vi "Open IPF.vi"(3 "Error In":errorcluster, 4 "?":T2) -> (0 "Error Out":errorcluster, 1 "IPF refnum":T1, 2 "IPF Path":path)   [LabVIEW 2018]
uses:
  Type Defs/Open IPF.ctl
  <vilib>/Utility/config.llb/Config Data RefNum.ctl
  <vilib>/Utility/config.llb/NI_LVConfig.lvlib
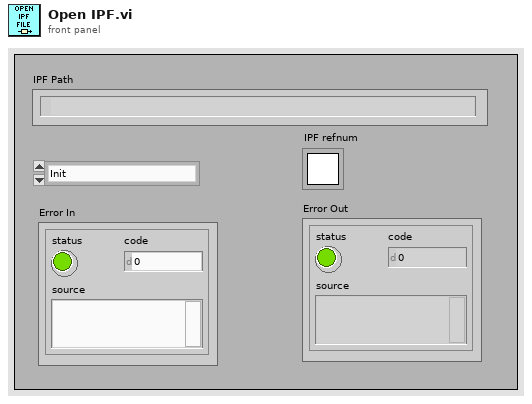
[diagram p1: front panel]
types:
  T1 = typedef "NI_LVConfig.lvlib/Config Data RefNum.ctl" = refnum<k1>
  T2 = typedef "Open IPF.ctl" = enum16{"Init", "Create IPF"}
  T3 = enum32{"existing file", "new file", "new or existing file", "existing dir", "new dir", "new or existing dir", "existing file (use LLBs)", "new file (use LLBs)", "new or existing file (use LLBs)", "new or existing file or directory (use LLBs)"}
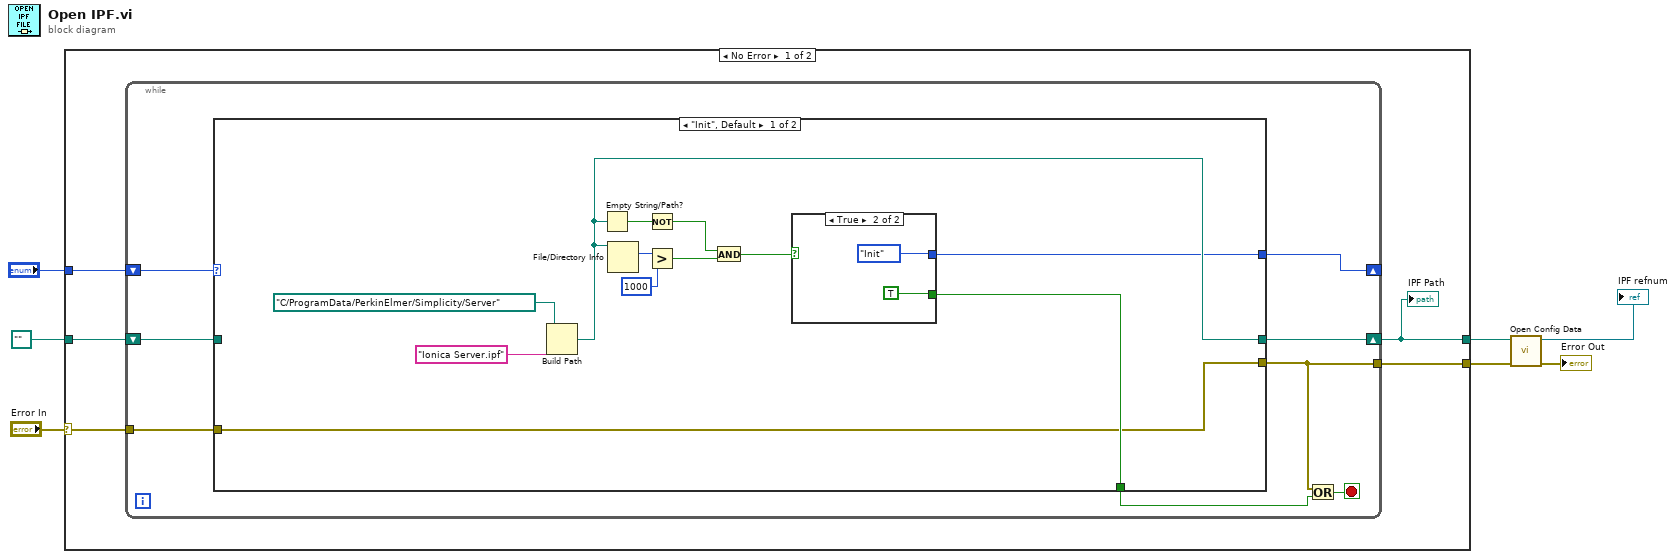
[diagram p0: block diagram]
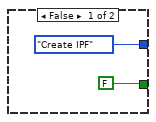
[diagram p2: hidden frame]
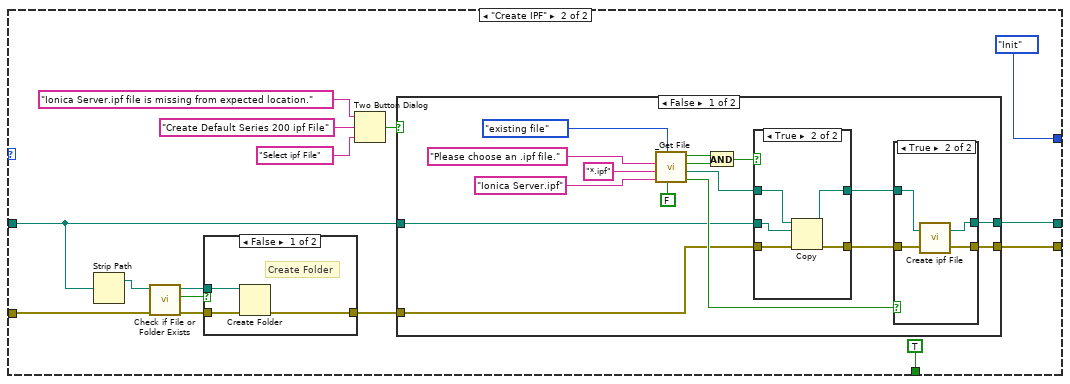
[diagram p3: hidden frame]
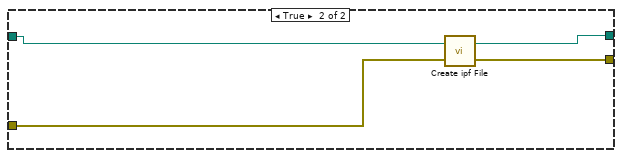
[diagram p6: hidden frame]
diagram:
  n1 = case shown="No Error" "Error In" {
    selector: "Error In" -> [w11 w90]
    tunnel: [w10 w90] -> w5
    tunnel: "?" -> [w12 _]
    tunnel: [w8 w89] -> w4
    tunnel: path "" ("ipf file path") -> [w9 w89]
    frame No Error {
      n2 = while {
        tunnel: w11 -> [w19]
        tunnel: [w15] -> w10
        shift-right: [w17] -> w8
        shift-left: w9 -> [w18]
        shift-right: [w13] -> _
        shift-left: w12 -> [w20]
        stop <- w16 stop-if-true
        n3 = case shown="\"Init\", Default" w20 {
          tunnel: w19 -> [w21 w44]
          tunnel: [w21 w39] -> w15
          tunnel: w18 -> [_ w42]
          tunnel: [w25 w40] -> w17
          tunnel: [w23 TRUE] -> w14
          tunnel: [w22 Open_IPF."Init"] -> w13
          frame "Init", Default {
            n4 = Build Path(base path=path "C:/ProgramData/PerkinElmer/Simplicity/Server" ("appended path"), name or relative path="Ionica Server.ipf") -> (appended path=w25:path)
            n5 = Empty String/Path?(string/path=w25) -> (empty?=w28:bool)
            n6 = File/Directory Info(path=w25) -> (size=w29:i64)  [unwired: 1 in, 6 out]
            n7 = Not(x=w28) -> (.not. x?=w26:bool)
            n8 = Greater?(x=w29, y=i64 1000) -> (0:w27:bool)
            n9 = And(x=w26, y=w27) -> (x .and. y?=w24:bool)
            n10 = case shown="True" w24 {
              tunnel: [FALSE TRUE] -> w23
              tunnel: [Open_IPF."Create IPF" Open_IPF."Init"] -> w22
              frame False {
              }
              frame True {
              }
            }
          }
          frame "Create IPF" {
            n11 = Strip Path(path=w42) -> (stripped path=w48:path)  [unwired: 1 out]
            n12 = call <vilib>:"Check if File or Folder Exists.vi"("error in (no error)"=w44, "path"=w48) -> ("error out"=w51:errorcluster, "file or folder exists?"=w49:bool, "dup path"=w50:path)  [unwired: 7 in]
            n13 = case shown="False" w49 {
              tunnel: w51 -> [w87 w88]
              tunnel: [w86 w88] -> w43
              tunnel: w50 -> [w85 _]
              frame False {
                # "Create Folder"
                n14 = Create Folder(path (use dialog)=w85, error in=w87) -> (error out=w86:errorcluster)  [unwired: 1 in, 2 out]
              }
              frame True {
              }
            }
            n15 = Two Button Dialog(message="Ionica Server.ipf file is missing from expected location.", 1:"Select ipf File" ("T button name (\"OK\")"), 2:"Create Default Series 200 ipf File" ("T button name (\"OK\")")) -> (T button?=w41:bool)
            n16 = case shown="False" w41 {
              tunnel: [w57 w84] -> w39
              tunnel: [w55 w81] -> w40
              tunnel: w43 -> [w52 w83]
              tunnel: w42 -> [w53 w82]
              frame False {
                n17 = call "_Get File.vi"("For Write (T)"=FALSE, "select mode (new or existing)"=T3."existing file", "default name"="Ionica Server.ipf", "extension (isd)"="*.ipf", "prompt"="Please choose an .ipf file.") -> ("cancelled"=w54:bool, "Seleted File"=w59:path, "Exists"=w61:bool, "Succeeded"=w62:bool)  [unwired: 1 in]
                n18 = And(x=w62, y=w61) -> (x .and. y?=w60:bool)
                n19 = case shown="True" w60 {
                  tunnel: w59 -> [_ w80]
                  tunnel: [w75 w79] -> w56
                  tunnel: [w74 w78] -> w58
                  tunnel: w53 -> [w75 w76]
                  tunnel: w52 -> [w74 w77]
                  frame False {
                  }
                  frame True {
                    n20 = Copy(8:w77, 10:w76, 11:w80) -> (0:w78:errorcluster, 3:w79:path)  [unwired: 2 in, 1 out]
                  }
                }
                n21 = case shown="True" w54 {
                  tunnel: w58 -> [w69 w73]
                  tunnel: [w69 w72] -> w57
                  tunnel: w56 -> [w68 w71]
                  tunnel: [w68 w70] -> w55
                  frame False {
                  }
                  frame True {
                    n22 = call "Create ipf File.vi"("error in"=w73, "Default ipf file path"=w71) -> ("error out"=w72:errorcluster, "ipf file path"=w70:path)
                  }
                }
              }
              frame True {
                n23 = call "Create ipf File.vi"("error in"=w83, "Default ipf file path"=w82) -> ("error out"=w84:errorcluster, "ipf file path"=w81:path)
              }
            }
          }
        }
        n24 = Or(x=w15, y=w14) -> (x .or. y?=w16:bool)
      }
      "IPF Path" <- w8
    }
    frame Error {
    }
  }
  n25 = call <vilib>:"Open Config Data.vi"("error in (no error)"=w5, "configuration file path"=w4) -> ("error out"=→"Error Out":errorcluster, "refnum"=→"IPF refnum":T1)  [unwired: 7 in, 1 out]
